vi "_FPGA_8bitsCountDownStrobe.vi"(9 "Count down":u8, 10 "Conj?":bool, 11 "Load":bool) -> (3 "terminal count strobe":bool)   [LabVIEW 2018]
uses:
  <instrlib>/_niInstr/Basic Elements/v1/FPGA/Private/Count Down U8.vi
  <instrlib>/_niInstr/Basic Elements/v1/FPGA/niInstr Basic Elements v1 FPGA.lvlib
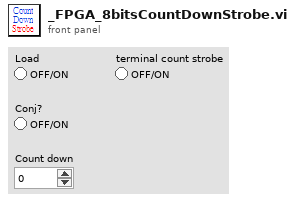
[diagram p1: front panel]
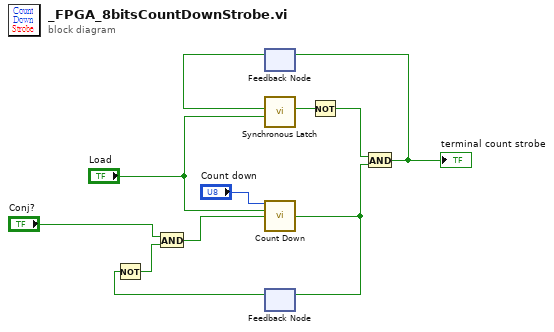
[diagram p0: block diagram]
diagram:
  n1 = feedback #1() -> (w2:bool)  [unwired: 1 in]
  n2 = call <instrlib>:"Synchronous Latch.vi"("clear"="Load", "set"=w2) -> ("out"=w4:bool)  [unwired: 9 in]
  n3 = feedback #2() -> (w10:bool)  [unwired: 1 in]
  n4 = Not(x=w10) -> (.not. x?=w9:bool)
  n5 = And(x="Conj?", y=w9) -> (x .and. y?=w11:bool)
  n6 = call-poly <instrlib>:"Count Down.vi"("count in"="Count down", "load"="Load", "decrement"=w11) -> ("terminal count"=w5:bool)  [unwired: 11 in, 1 out]
  n7 = feedback-in #2(w5) -> ()
  n8 = Not(x=w4) -> (.not. x?=w3:bool)
  n9 = And(x=w3, y=w5) -> (x .and. y?=w1:bool)
  "terminal count strobe" <- w1
  n10 = feedback-in #1(w1) -> ()
